vi "Lector_Ingen.vi"() -> ()   [LabVIEW 2017]
uses:
  <vilib>/NI Modbus.llb/MB Ethernet Master Query Read Holding Registers (poly).vi
  <vilib>/NI Modbus.llb/MB Ethernet Master Query Write Multiple Registers (poly).vi
panel:
  in  "Tab Control 2":T1(tab)
  in  "CONTROL TEMPERATURA":cluster{"SET POINT":dbl, "INC T":dbl}
  out "TEMPERATURA ACTUAL":dbl
  in  "CONTROL DE PRESIÓN":cluster{"SET POINT":dbl, "INC P":dbl}
  out "PRESIÓN ACTUAL":dbl
  in  "CONTROL DE HUMEDAD":cluster{"SET POINT":dbl, "INC %":dbl}
  out "HUMEDAD ACTUAL":dbl
  in  "CONTROL DE LLENADO":cluster{"SET POINT":dbl, "INC  L":dbl}
  out "VOLUMEN ACTUAL":dbl
  out "Holding Registers":u16[](array[numeric])
  out "error out":errorcluster
  in  "Stop":bool
  in  "address":string="localhost"
  in  "Tab Control":T2(tab)
  out "Voltaje Fase 3":dbl(graph)
  out "Voltaje Fase 2":dbl(graph)
  out "Voltaje Fase 1":dbl(graph)
  out "Voltaje Promedio":dbl(graph)
  out "Corriente Promedio":dbl(graph)
  out "Corriente Fase 1":dbl(graph)
  out "Corriente Fase 2":dbl(graph)
  out "Corriente Fase 3":dbl(graph)
  out "Potencia Fase 3":dbl(graph)
  out "Potencia Fase 2":dbl(graph)
  out "Potencia Fase 1":dbl(graph)
  out "Potencia Promedio":dbl(graph)
  out "Factor de Potencia Fase 3":dbl(graph)
  out "Factor de Potencia Fase 2":dbl(graph)
  out "Factor de Potencia Fase 1":dbl(graph)
  out "Factor de Potencia Promedio":dbl(graph)
  out "Frecuencia":dbl(graph)
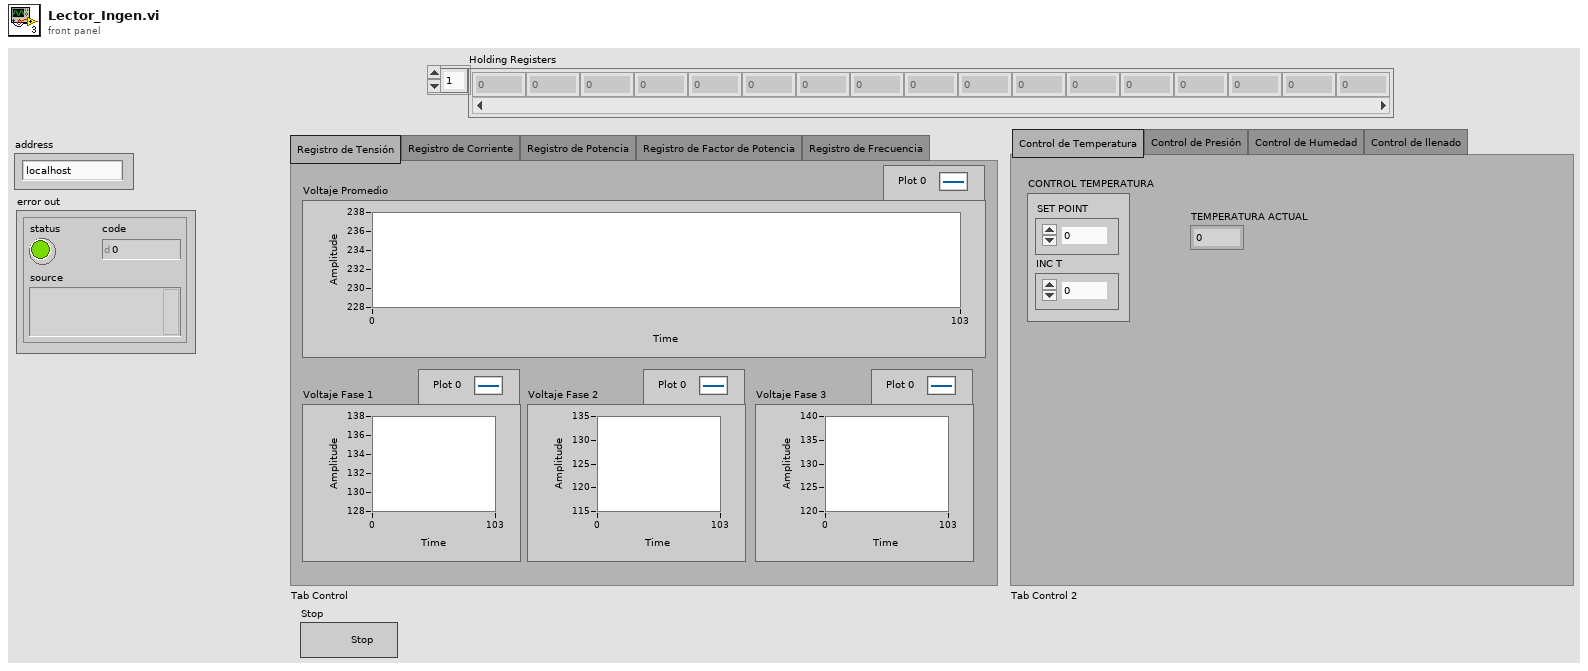
[diagram p1: front panel]
types:
  T1 = enum32{"Control de Temperatura", "Control de Presión", "Control de Humedad", "Control de llenado"}
  T2 = enum32{"Registro de Tensión", "Registro de Corriente", "Registro de Potencia", "Registro de Factor de Potencia", "Registro de Frecuencia"}
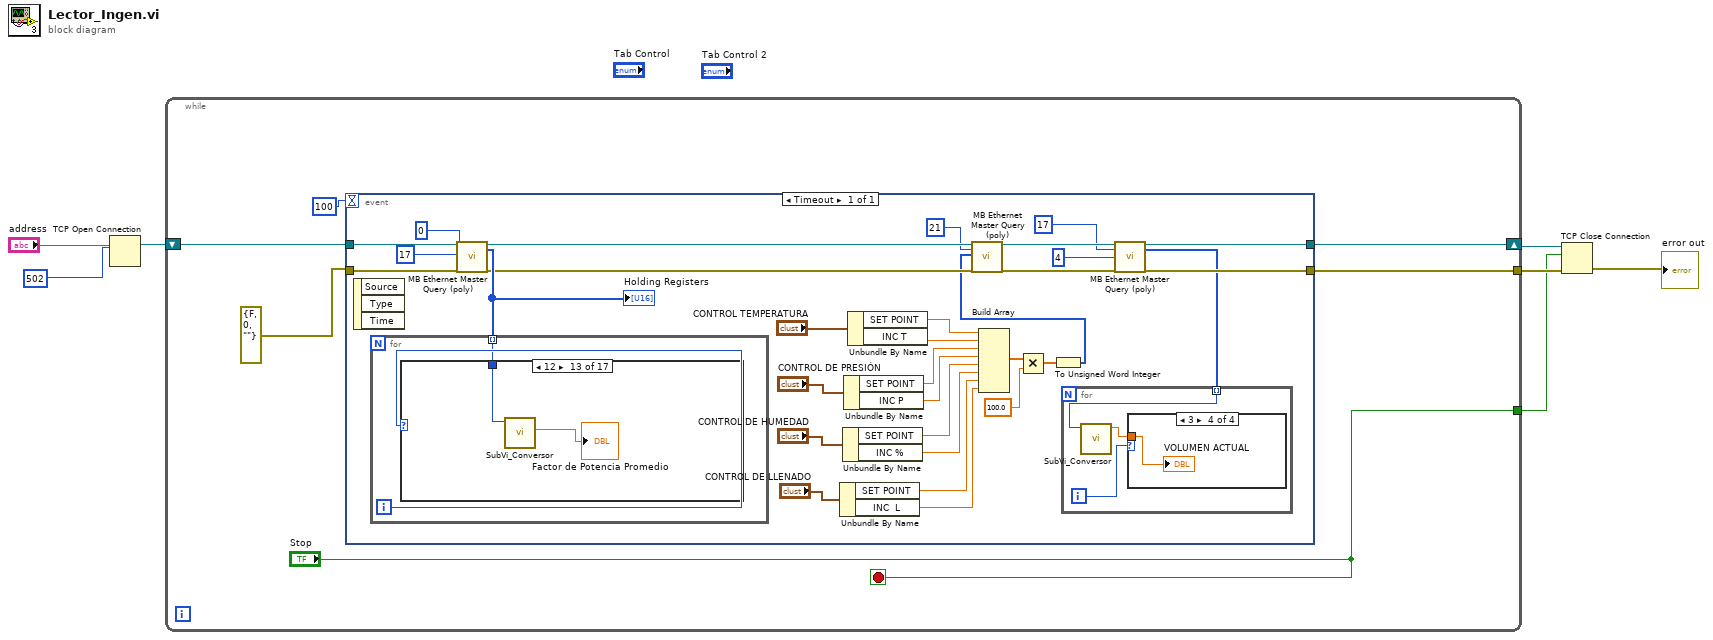
[diagram p0: block diagram]
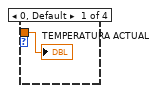
[diagram p2: hidden frame]
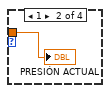
[diagram p3: hidden frame]
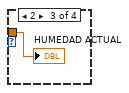
[diagram p4: hidden frame]
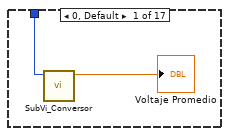
[diagram p5: hidden frame]
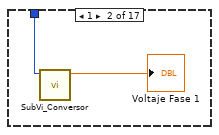
[diagram p6: hidden frame]
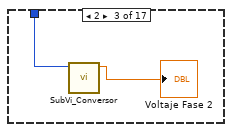
[diagram p7: hidden frame]
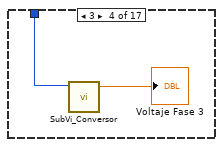
[diagram p8: hidden frame]
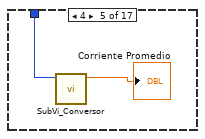
[diagram p9: hidden frame]
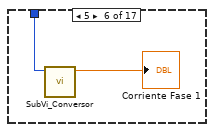
[diagram p10: hidden frame]
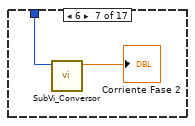
[diagram p11: hidden frame]
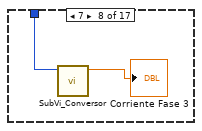
[diagram p12: hidden frame]
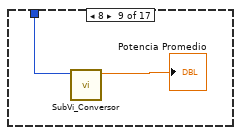
[diagram p13: hidden frame]
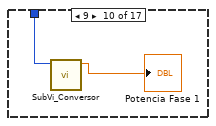
[diagram p14: hidden frame]
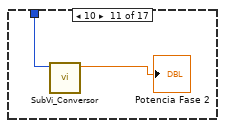
[diagram p15: hidden frame]
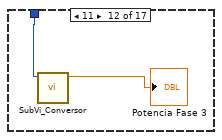
[diagram p16: hidden frame]
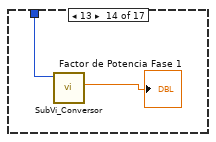
[diagram p17: hidden frame]
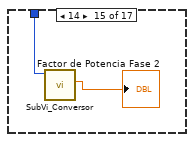
[diagram p18: hidden frame]
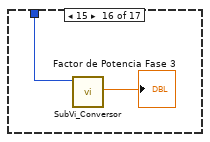
[diagram p19: hidden frame]
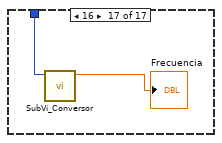
[diagram p20: hidden frame]
diagram:
  n1 = TCP Open Connection(address="address", remote port or service name=u16 502) -> (connection ID=w5:refnum<k5>)  [unwired: 3 in, 1 out]
  n2 = while {
    tunnel: [w11] -> w3
    shift-right: [w12] -> w4
    shift-left: w5 -> [w10]
    tunnel: ["Stop"] -> w2
    stop <- "Stop" stop-if-true
    n3 = event shown="[0] Timeout" {
      selector: _ -> [_]
      dyn-events: _ -> [_]
      timeout: 100 -> [_]
      tunnel: w10 -> [w44]
      tunnel: errorcluster {"status"=FALSE, "code"=0, "source"=""} ("error out") -> [w43]
      tunnel: [w16] -> w12
      tunnel: [w15] -> w11
      event Timeout {
        n4 = event-data() -> ()  [unwired: 1 in, 3 out]
        n5 = call-poly <vilib>:"MB Ethernet Master Query (poly).vi"("TCP Connection Refnum in"=w44, "Starting Address"=u16 0, "Quantity"=u16 17, "error in"=w43) -> ("TCP Connection Refnum (dup)"=w24:refnum<k5>, "Holding Registers"=w40:u16[], "error out"=w23:errorcluster)  [unwired: 12 in, 1 out]
        "Holding Registers" <- w40
        n6 = for {
          tunnel: w40 -> [w52] mode=indexing
          i -> [w53]
          n7 = case shown="12" w53 {
            tunnel: w52 -> [w55 w56 w59 w60 w63 w65 w67 w69 w71 w73 w75 w76 w78 w81 w83 w84 w86]
            frame 0, Default {
              n8 = call "SubVi_Conversor.vi"("Entrada_U16"=w55) -> ("Dato"=→"Voltaje Promedio":dbl)  [unwired: 9 in, 1 out]
            }
            frame 1 {
              n9 = call "SubVi_Conversor.vi"("Entrada_U16"=w56) -> ("Dato"=→"Voltaje Fase 1":dbl)  [unwired: 9 in, 1 out]
            }
            frame 2 {
              n10 = call "SubVi_Conversor.vi"("Entrada_U16"=w59) -> ("Dato"=→"Voltaje Fase 2":dbl)  [unwired: 9 in, 1 out]
            }
            frame 3 {
              n11 = call "SubVi_Conversor.vi"("Entrada_U16"=w60) -> ("Dato"=→"Voltaje Fase 3":dbl)  [unwired: 9 in, 1 out]
            }
            frame 4 {
              n12 = call "SubVi_Conversor.vi"("Entrada_U16"=w63) -> ("Dato"=→"Corriente Promedio":dbl)  [unwired: 9 in, 1 out]
            }
            frame 5 {
              n13 = call "SubVi_Conversor.vi"("Entrada_U16"=w65) -> ("Dato"=→"Corriente Fase 1":dbl)  [unwired: 9 in, 1 out]
            }
            frame 6 {
              n14 = call "SubVi_Conversor.vi"("Entrada_U16"=w67) -> ("Dato"=→"Corriente Fase 2":dbl)  [unwired: 9 in, 1 out]
            }
            frame 7 {
              n15 = call "SubVi_Conversor.vi"("Entrada_U16"=w69) -> ("Dato"=→"Corriente Fase 3":dbl)  [unwired: 9 in, 1 out]
            }
            frame 8 {
              n16 = call "SubVi_Conversor.vi"("Entrada_U16"=w71) -> ("Dato"=→"Potencia Promedio":dbl)  [unwired: 9 in, 1 out]
            }
            frame 9 {
              n17 = call "SubVi_Conversor.vi"("Entrada_U16"=w73) -> ("Dato"=→"Potencia Fase 1":dbl)  [unwired: 9 in, 1 out]
            }
            frame 10 {
              n18 = call "SubVi_Conversor.vi"("Entrada_U16"=w75) -> ("Dato"=→"Potencia Fase 2":dbl)  [unwired: 9 in, 1 out]
            }
            frame 11 {
              n19 = call "SubVi_Conversor.vi"("Entrada_U16"=w76) -> ("Dato"=→"Potencia Fase 3":dbl)  [unwired: 9 in, 1 out]
            }
            frame 12 {
              n20 = call "SubVi_Conversor.vi"("Entrada_U16"=w78) -> ("Factor_de_potencia"=→"Factor de Potencia Promedio":dbl)  [unwired: 9 in, 1 out]
            }
            frame 13 {
              n21 = call "SubVi_Conversor.vi"("Entrada_U16"=w81) -> ("Factor_de_potencia"=→"Factor de Potencia Fase 1":dbl)  [unwired: 9 in, 1 out]
            }
            frame 14 {
              n22 = call "SubVi_Conversor.vi"("Entrada_U16"=w83) -> ("Factor_de_potencia"=→"Factor de Potencia Fase 2":dbl)  [unwired: 9 in, 1 out]
            }
            frame 15 {
              n23 = call "SubVi_Conversor.vi"("Entrada_U16"=w84) -> ("Factor_de_potencia"=→"Factor de Potencia Fase 3":dbl)  [unwired: 9 in, 1 out]
            }
            frame 16 {
              n24 = call "SubVi_Conversor.vi"("Entrada_U16"=w86) -> ("Dato"=→"Frecuencia":dbl)  [unwired: 9 in, 1 out]
            }
          }
        }
        n25 = Unbundle By Name("CONTROL DE LLENADO") -> ("SET POINT"=w29:dbl, "INC  L"=w28:dbl)
        n26 = Unbundle By Name("CONTROL DE HUMEDAD") -> ("SET POINT"=w31:dbl, "INC %"=w30:dbl)
        n27 = Unbundle By Name("CONTROL DE PRESIÓN") -> ("SET POINT"=w33:dbl, "INC P"=w32:dbl)
        n28 = Unbundle By Name("CONTROL TEMPERATURA") -> ("SET POINT"=w35:dbl, "INC T"=w34:dbl)
        n29 = Build Array(w35, w34, w33, w32, w31, w30, w29, w28) -> (w27:dbl[])
        n30 = Multiply(x=w27, y=100.0) -> (x*y=w25:dbl[])
        n31 = To Unsigned Word Integer(number=w25) -> (unsigned 16bit integer=w21:u16[])
        n32 = call-poly <vilib>:"MB Ethernet Master Query (poly).vi"("TCP Connection Refnum in"=w24, "Starting Address"=u16 21, "Registers"=w21, "error in"=w23) -> ("TCP Connection Refnum (dup)"=w20:refnum<k5>, "error out"=w19:errorcluster)  [unwired: 13 in, 1 out]
        n33 = call-poly <vilib>:"MB Ethernet Master Query (poly).vi"("TCP Connection Refnum in"=w20, "Starting Address"=u16 17, "Quantity"=u16 4, "error in"=w19) -> ("TCP Connection Refnum (dup)"=w16:refnum<k5>, "Holding Registers"=w14:u16[], "error out"=w15:errorcluster)  [unwired: 12 in, 1 out]
        n34 = for {
          tunnel: w14 -> [w47] mode=indexing
          i -> [w46]
          n35 = call "SubVi_Conversor.vi"("Entrada_U16"=w47) -> ("Dato"=w45:dbl)  [unwired: 9 in, 1 out]
          n36 = case shown="3" w46 {
            tunnel: w45 -> [w48 w49 w50 w51]
            frame 0, Default {
              "TEMPERATURA ACTUAL" <- w48
            }
            frame 1 {
              "PRESIÓN ACTUAL" <- w49
            }
            frame 2 {
              "HUMEDAD ACTUAL" <- w50
            }
            frame 3 {
              "VOLUMEN ACTUAL" <- w51
            }
          }
        }
      }
    }
  }
  n37 = TCP Close Connection(connection ID=w4, abort (F)=w2, error in (no error)=w3) -> (error out=→"error out":errorcluster)  [unwired: 1 out]
